vi "Read SIMULATED_ TI.vi"(8 "error in (no error)":errorcluster, 11 "TI in":refnum<class "TI.lvclass">) -> (0 "error out":errorcluster, 2 "SIMULATED?":bool, 3 "TI out":refnum<class "TI.lvclass">)   [LabVIEW 2019, in "TI.lvclass"]
uses:
  TI.lvclass
  TI.lvclass/TI.ctl
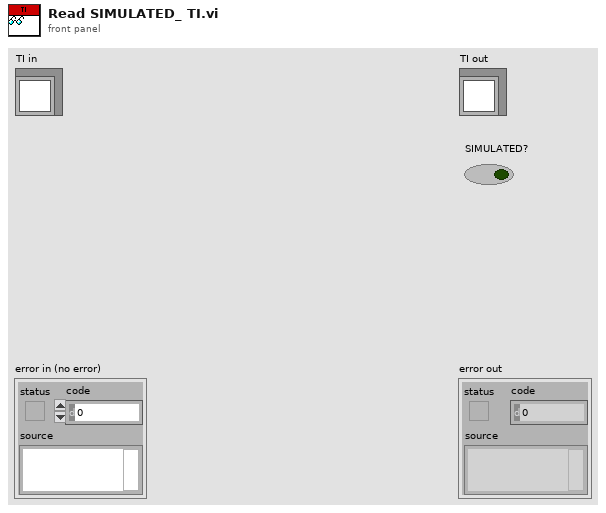
[diagram p1: front panel]
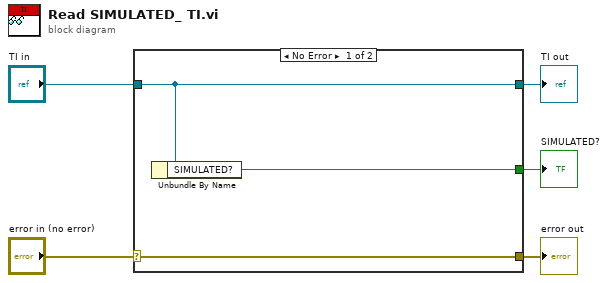
[diagram p0: block diagram]
diagram:
  n1 = case shown="No Error" "error in (no error)" {
    selector: "error in (no error)" -> [w8 w9]
    tunnel: [w8 w9] -> w4
    tunnel: [w7 w10] -> w2
    tunnel: "TI in" -> [w7 w10]
    tunnel: [w6 _] -> w1
    frame No Error {
      n2 = Unbundle By Name(w7) -> ("SIMULATED?"=w6:bool)
    }
    frame Error {
    }
  }
  "error out" <- w4
  "TI out" <- w2
  "SIMULATED?" <- w1
